vi "Test_ReadValue_NeverWritten_TimeoutError.vi"(8 "error in (no error)":errorcluster, 11 "TestCase in":refnum<class "TestNotifierTransport.lvclass">) -> (0 "error out":errorcluster, 3 "TestCase out":refnum<class "TestNotifierTransport.lvclass">)   [LabVIEW 2017, in "TestNotifierTransport.lvclass"]
uses:
  TestNotifierTransport.lvclass
  Source/Concrete/NotifierTransport/NotifierTransport.lvclass/NotifierTransport.ctl
  <vilib>/Utility/error.llb/Error Cluster From Error Code.vi
  Source/Concrete/NotifierTransport/NotifierTransport.lvclass
panel:
  out "Return Error":errorcluster
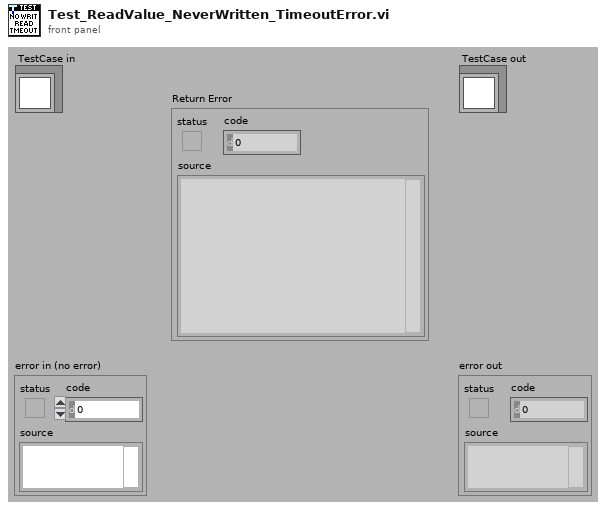
[diagram p1: front panel]
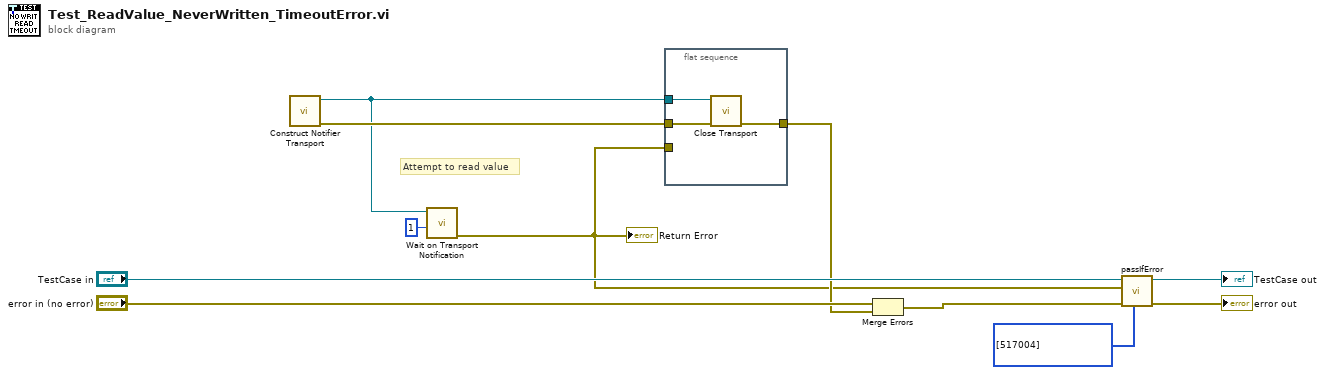
[diagram p0: block diagram]
diagram:
  # "Attempt to read value"
  n1 = call "Construct Notifier Transport.vi"() -> ("error out"=w4:errorcluster, "NotifierTransport"=w1:refnum<class "NotifierTransport.lvclass">)  [unwired: 10 in]
  n2 = call "Wait on Transport Notification.vi"("Timeout In ms (-1)"=1, "NotifierTransport"=w1) -> ("error out"=w2:errorcluster)  [unwired: 7 in, 2 out]
  "Return Error" <- w2
  n3 = flat-sequence {
    tunnel: w4 -> [w14]
    tunnel: [w13] -> w3
    tunnel: w1 -> [w12]
    tunnel: w2 -> [_]
    frame #0 {
      n4 = call-dynamic "Close Transport.vi"("error in (no error)"=w14, "NotifierTransport"=w12) -> ("error out"=w13:errorcluster)  [unwired: 9 in]
    }
  }
  n5 = Merge Errors("error in (no error)", w3) -> (w6:errorcluster)
  n6 = call-dynamic "passIfError.vi"("passing error codes (default = any error code)"=i32[] [517004], "error in (no error)"=w6, "error"=w2, "TestCase in"="TestCase in") -> ("error out"=→"error out":errorcluster, "TestCase out"=→"TestCase out":refnum<class "TestNotifierTransport.lvclass">)  [unwired: 6 in]
